vi "Set All Joint Positions.vi"(6 "Coordinate Space":enum16{"Color Space", "Depth Space"}(ring), 8 "error in (no error)":errorcluster, 9 "Body Index":i32, 10 "Joints":refnum<k24>, 11 "KinectSensor Reference":refnum<k24>) -> (0 "error out":errorcluster)   [LabVIEW 2014]
uses:
  Microsoft.Kinect
  controls/JointType.ctl
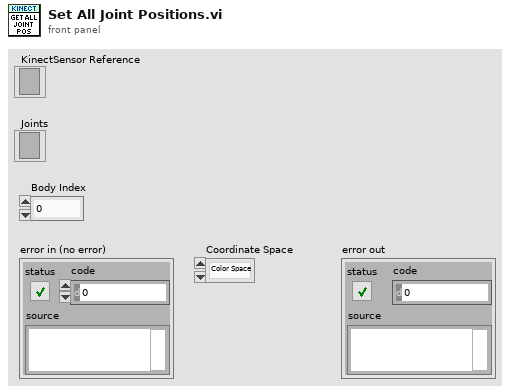
[diagram p1: front panel]
types:
  T1 = enum16{"Get Joint Position", "Initialize", "Set Joint Position"}
  T2 = typedef "JointType.ctl" = i32
  T3 = typedef "Joint Position.ctl" = cluster{"Position":cluster{"X":sgl, "Y":sgl}, "TrackingState":i32}
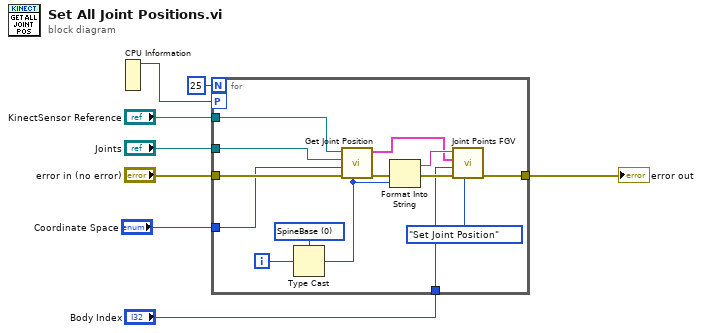
[diagram p0: block diagram]
diagram:
  n1 = CPU Information() -> (4:w1:i32)  [unwired: 3 out]
  n2 = for {
    N: 25 -> [_]
    tunnel: "KinectSensor Reference" -> [w18]
    tunnel: "Joints" -> [w19]
    tunnel: "Coordinate Space" -> [w11]
    tunnel: "error in (no error)" -> [w20]
    tunnel: [w12] -> w3
    workers-P: w1 -> [_]
    tunnel: "Body Index" -> [w9]
    i -> [w22]
    w21 = T2 0 items=["SpineBase", "SpineMid", "Neck", "Head", "ShoulderLeft", "ElbowLeft", "WristLeft", "HandLeft", "ShoulderRight", "ElbowRight", "WristRight", "HandRight", "HipLeft", "KneeLeft", "AnkleLeft", "FootLeft", "HipRight", "KneeRight", "AnkleRight", "FootRight", "SpineShoulder", "HandTipLeft", "ThumbLeft", "HandTipRight", "ThumbRight"] ("JointType")
    n3 = Type Cast(type=w21, x=w22) -> (*(type *) &x=w14:T2)
    n4 = call "Get Joint Position.vi"("JointType"=w14, "error in (no error)"=w20, "Coordinate Space"=w11, "Joints"=w19, "KinectSensor Reference"=w18) -> ("error out"=w15:errorcluster, "Joint Position"=w13:T3)  [unwired: 5 in]
    n5 = Format Into String(error in=w15, w14) -> (resulting string=w17:string, error out=w16:errorcluster)  [unwired: 2 in]
    n6 = call "Joint Points FGV.vi"("Command"=T1."Set Joint Position", "error in (no error)"=w16, "Body Index"=w9, "Joint Position"=w13, "name"=w17) -> ("error out"=w12:errorcluster)  [unwired: 5 in, 1 out]
  }
  "error out" <- w3
